vi "SDG60ConfPRBS.vi"(2 "Differental mode (0: Off)":u16(ring) items=["Off", "On"], 4 "Offset (0.00 V)":dbl min=-10.0 max=10.0 format="%#_15g", 5 "BitRate/Period (T:BitRate)":bool=TRUE, 6 "Amplitude (1 Vpp)":dbl=1.0, 7 "Length (3)":u16=3, 9 "Bit Rate/Period (1000 bits/second)":dbl=1000.0 format="%#_15g", 10 "Channel (1: Ch1)":u16(ring)=1 items=["Channel 1"=1, "Channel 2"=2]) -> ()   [LabVIEW 2022 SP3]
doc: "Configures PRBS waveform and parameters.\n\nNote:\nThis VI only supports SDG6000X series."
uses:
  <vilib>/addons/zeromq/socket_type.ctl
  <vilib>/addons/zeromq/zmq_context.lvclass
  <vilib>/addons/zeromq/zmq_socket.lvclass
  <vilib>/addons/zeromq/zeromq.lvlib
panel:
  out "Python response":string
  in  "Instrument Gen":string
  in  "Edge Time (10 ns)":dbl=1e-08 format="%#_16g"
  # "Logic Level changable only via front panel"
  # "Range 1 mbit/sec to 300 Mbits/sec\n10 digits precision"
  # "Range: 3-32\nActual PRBS length = 2^(LENGTH)-1"
  # "Range:1ns - 1ms Max depends on period\n6 digits precision"
  # "Range: 2mVpp-20Vpp\n6 digits precision"
  # "Range +/- 9.999V\n6 digits precision"
  # "Will be really differential when both ch\noutputs are ON. Switching outputs OFF ruins phase relation of the channels"
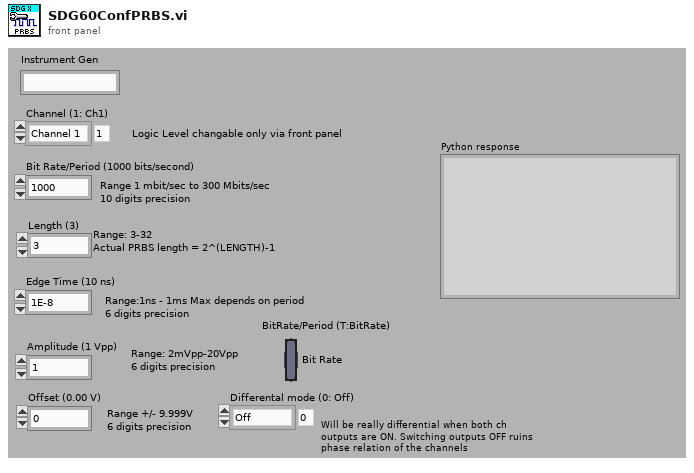
[diagram p1: front panel]
types:
  T1 = typedef "zeromq.lvlib/socket_type.ctl" = enum8{"ZMQ_PAIR", "ZMQ_PUB", "ZMQ_SUB", "ZMQ_REQ", "ZMQ_REP", "ZMQ_DEALER", "ZMQ_ROUTER", "ZMQ_PULL", "ZMQ_PUSH", "ZMQ_XPUB", "ZMQ_XSUB", "ZMQ_STREAM", "ZMQ_SERVER", "ZMQ_CLIENT", "ZMQ_RADIO", "ZMQ_DISH", "ZMQ_GATHER", "ZMQ_SCATTER", "ZMQ_DGRAM"}
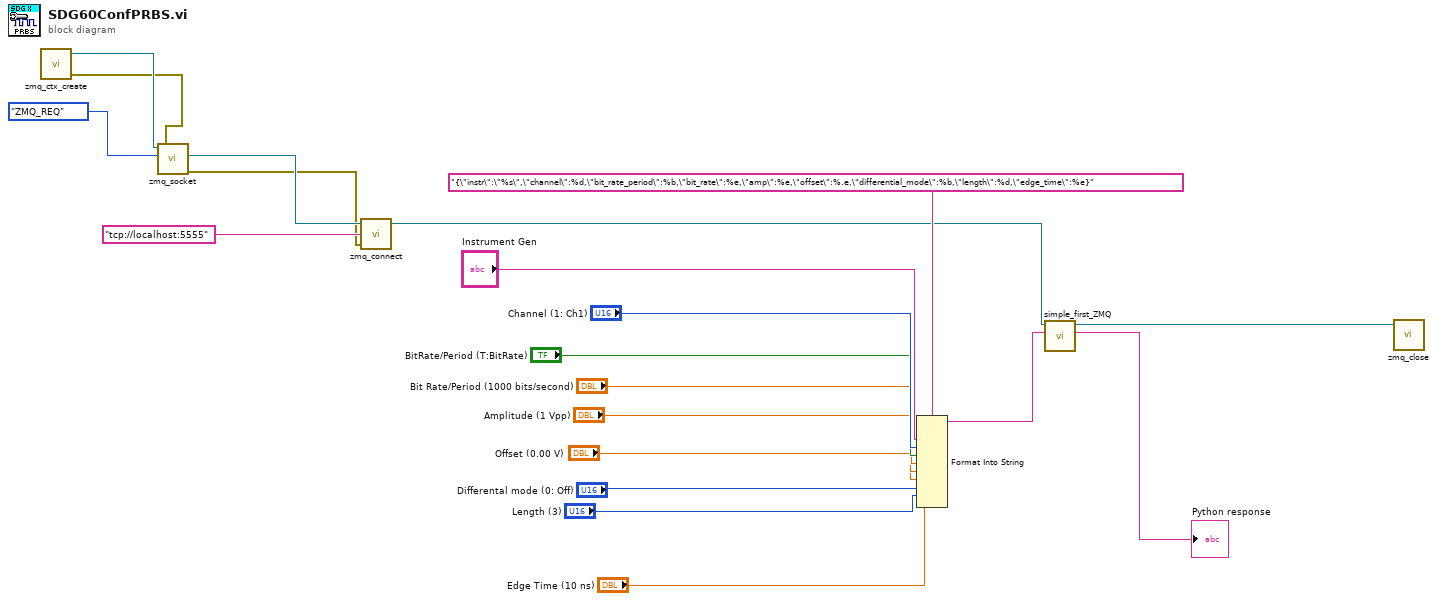
[diagram p0: block diagram]
diagram:
  n1 = call <vilib>:"zmq_ctx_create.vi"() -> ("error out"=w7:errorcluster, "context out"=w9:refnum<class "zmq_context.lvclass">)  [unwired: 4 in]
  n2 = call <vilib>:"zmq_socket.vi"("error in"=w7, "socket type"=socket_type."ZMQ_REQ", "context in"=w9) -> ("error out"=w4:errorcluster, "socket out"=w8:refnum<class "zmq_socket.lvclass">)  [unwired: 2 in, 1 out]
  n3 = call <vilib>:"zmq_connect.vi"("error in"=w4, "endpoint"="tcp://localhost:5555", "socket in"=w8) -> ("socket out"=w3:refnum<class "zmq_socket.lvclass">)  [unwired: 1 in, 1 out]
  n4 = Format Into String(format string="{\"instr\":\"%s\",\"channel\":%d,\"bit_rate_period\":%b,\"bit_rate\":%e,\"amp\":%e,\"offset\":%.e,\"differential_mode\":%b,\"length\":%d,\"edge_time\":%e}", "Instrument Gen", "Channel (1: Ch1)", "BitRate/Period (T:BitRate)", "Bit Rate/Period (1000 bits/second)", "Amplitude (1 Vpp)", "Offset (0.00 V)", "Differental mode (0: Off)", "Length (3)", "Edge Time (10 ns)") -> (resulting string=w10:string)  [unwired: 2 in, 1 out]
  n5 = call "simple_first_ZMQ.vi"("Raw command"=w10, "ZMQ socket in"=w3) -> ("Python response"=→"Python response":string, "ZMQ socket out"=w2:refnum<class "zmq_socket.lvclass">)  [unwired: 4 in]
  n6 = call <vilib>:"zmq_close.vi"("socket"=w2) -> ()  [unwired: 4 in, 1 out]
